vi "Set AO Sampling Rate.vi"(8 "error in (no error)":errorcluster, 9 "Fs (Hz)":dbl, 11 "Tosca in":refnum<class "Parameters.lvclass">) -> (0 "error out":errorcluster, 3 "Tosca out":refnum<class "Parameters.lvclass">)   [LabVIEW 2020, in "Parameters.lvclass"]
uses:
  Parameters.lvclass
  Parameters.lvclass/Parameters.ctl
  State/State.lvclass/State.ctl
  epl-vi-lib/Signal Synthesis VIs/4th Generation/Classes/SignalManager/SignalManager.lvclass/SignalManager.ctl
  State/Read SigMan.vi
  epl-vi-lib/Signal Synthesis VIs/4th Generation/Classes/SignalManager/Write Fs (Hz).vi
  State/Write SigMan.vi
  epl-vi-lib/Signal Synthesis VIs/4th Generation/Classes/SignalManager/SignalManager.lvclass
  State/State.lvclass
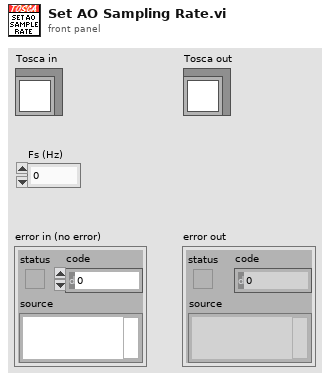
[diagram p1: front panel]
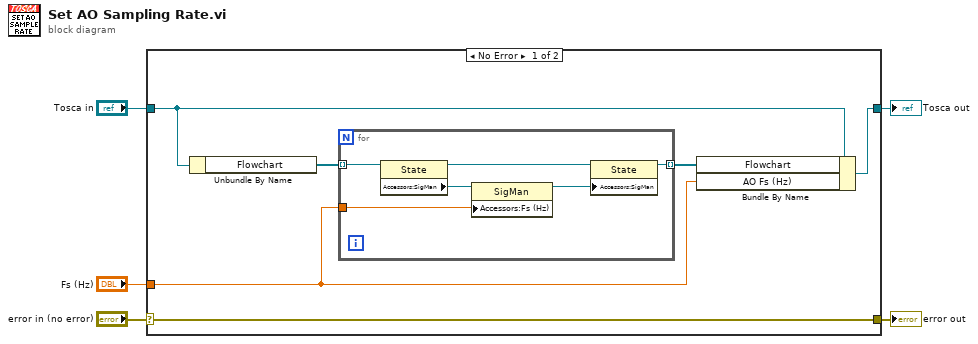
[diagram p0: block diagram]
diagram:
  n1 = case shown="No Error" "error in (no error)" {
    selector: "error in (no error)" -> [w11 w19]
    tunnel: [w11 w19] -> w4
    tunnel: [w8 w18] -> w2
    tunnel: "Tosca in" -> [w10 w18]
    tunnel: "Fs (Hz)" -> [w6 _]
    frame No Error {
      n2 = Unbundle By Name(w10) -> ("Flowchart"=w9:refnum<class "State.lvclass">[])
      n3 = for {
        tunnel: w9 -> [w17] mode=indexing
        tunnel: [w13] -> w7 mode=indexing
        tunnel: w6 -> [w12]
        n4 = property class="State"(reference=w17) -> (reference out=w15:refnum<class "State.lvclass">, "Accessors:SigMan"=w16:refnum<class "SignalManager.lvclass">)  [unwired: 1 in, 1 out]
        n5 = property class="SigMan"(reference=w16, "Accessors:Fs (Hz)"=w12) -> (reference out=w14:refnum<class "SignalManager.lvclass">)  [unwired: 1 in, 1 out]
        n6 = property class="State"(reference=w15, "Accessors:SigMan"=w14) -> (reference out=w13:refnum<class "State.lvclass">)  [unwired: 1 in, 1 out]
      }
      n7 = Bundle By Name(cluster=w10, "Flowchart"=w7, "AO Fs (Hz)"=w6) -> (w8:refnum<class "Parameters.lvclass">)
    }
    frame Error {
    }
  }
  "error out" <- w4
  "Tosca out" <- w2
